vi "Arange_Displays_V2.vi"(0 "Display References":refnum<vi>[](array[refnum]), 2 "Action":u16(ring) items=["Read", "Write"], 7 "Number of Channels":i32, 11 "Aspect Ratio (h/w)":dbl) -> (8 "Number of Channels OUT":i32)   [LabVIEW 2014]
uses:
  <vilib>/Utility/miscctls.llb/LVPositionTypeDef.ctl
  <vilib>/Utility/miscctls.llb/LVBoundsTypeDef.ctl
panel:
  in  "Display Number":i32=2
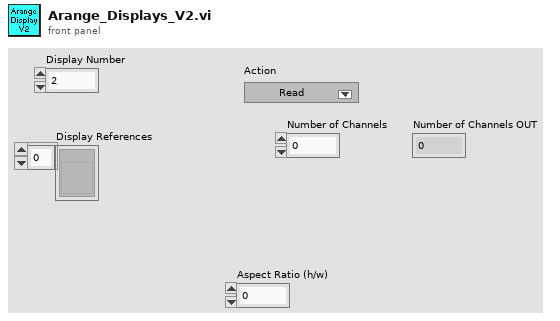
[diagram p1: front panel]
types:
  T1 = typedef "LVPositionTypeDef.ctl" = cluster{"Left":i32, "Top":i32}
  T2 = typedef "LVBoundsTypeDef.ctl" = cluster{"Width":u32, "Height":u32}
  T3 = typedef "LVAllMonitorsDisplayTypeDef.ctl" = cluster{"Bounds":cluster{"Left":i16, "Top":i16, "Right":i16, "Bottom":i16}, "Depth":i16}[]
  T4 = cluster{"Bounds":cluster{"Left":i16, "Top":i16, "Right":i16, "Bottom":i16}, "Depth":i16}
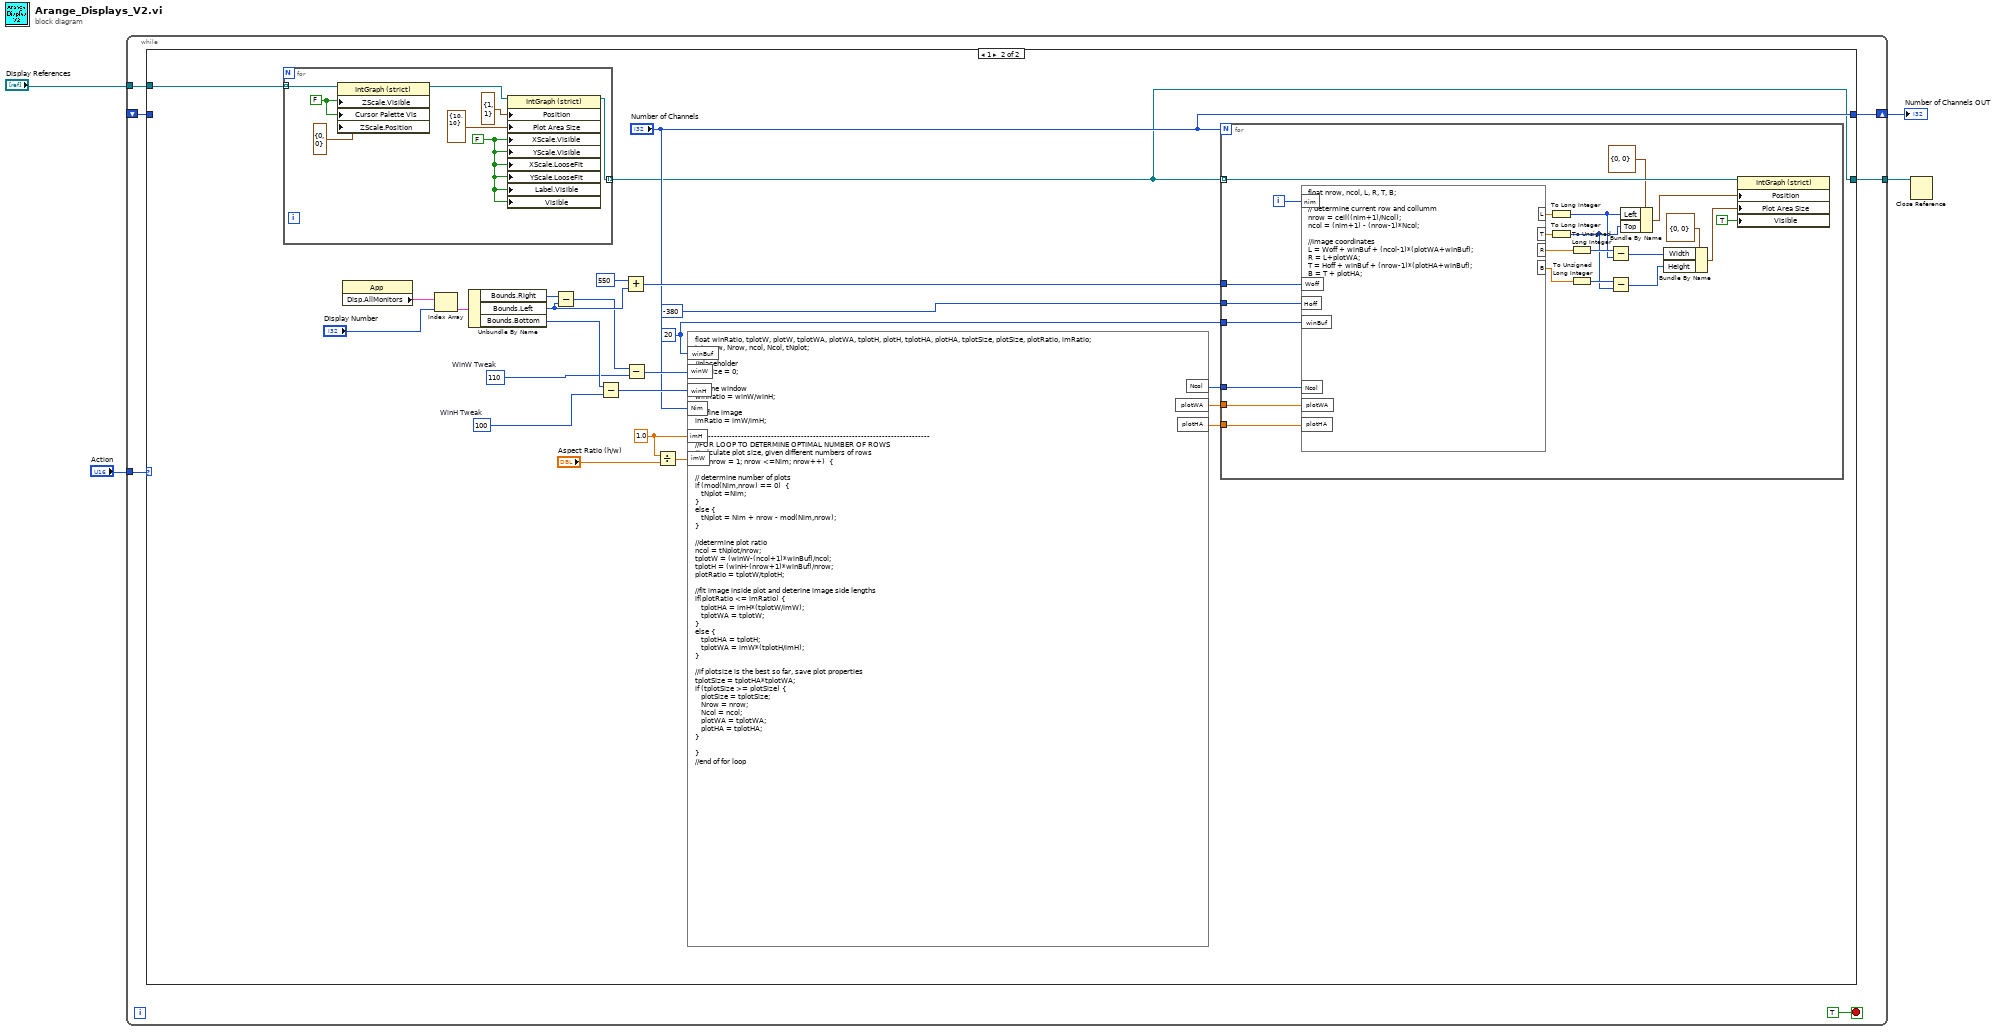
[diagram p0: block diagram]
diagram:
  n1 = while {
    tunnel: "Action" -> [w9]
    shift-right: [w8] -> w3
    shift-left: _ -> [w7]
    tunnel: "Display References" -> [w6]
    tunnel: [w5] -> w1
    stop <- TRUE stop-if-true
    n2 = case shown="1" w9 {
      tunnel: [w12 "Number of Channels"] -> w8
      tunnel: w7 -> [w12 _]
      tunnel: w6 -> [w11 w14]
      tunnel: [w11 w13] -> w5
      frame 0, Default {
      }
      frame 1 {
        w36 = 20 ("WinBuffer")
        w19 = i16 110  # WinW Tweak
        w22 = i16 100  # WinH Tweak
        w16 = 1.0 ("y")
        n3 = for {
          tunnel: [w41] -> w13 mode=indexing
          tunnel: w14 -> [w37] mode=indexing
          w38 = FALSE ("Z Scale.Visible")
          w42 = FALSE ("X Scale.Visible")
          n4 = property class="IntGraph (strict)"(reference=w37, "ZScale.Visible"=w38, "Cursor Palette Vis"=w38, "ZScale.Position"=T1 {"Left"=0, "Top"=0} ("Z Scale.Position")) -> (reference out=w40:refnum<vi>)  [unwired: 1 in, 1 out]
          n5 = property class="IntGraph (strict)"(reference=w40, "Position"=T1 {"Left"=1, "Top"=1}, "Plot Area Size"=T2 {"Width"=10, "Height"=10} ("Plot Area:Size"), "XScale.Visible"=w42, "YScale.Visible"=w42, "XScale.LooseFit"=w42, "YScale.LooseFit"=w42, "Label.Visible"=w42, "Visible"=w42) -> (reference out=w41:refnum<vi>)  [unwired: 1 in, 1 out]
        }
        n6 = property class="App"() -> ("Disp.AllMonitors"=w25:T3)  [unwired: 2 in, 2 out]
        n7 = Index Array(array=w25, index="Display Number") -> (element=w31:T4)
        n8 = Unbundle By Name(w31) -> ("Bounds.Right"=w28:i16, "Bounds.Left"=w27:i16, "Bounds.Bottom"=w24:i16)
        n9 = Subtract(x=w28, y=w27) -> (x-y=w21:i16)
        n10 = Subtract(x=w24, y=w22) -> (x-y=w23:i16)
        n11 = Add(x=i16 550 ("Woff"), y=w27) -> (x+y=w26:i16)
        n12 = Subtract(x=w21, y=w19) -> (x-y=w20:i16)
        n13 = Divide(x=w16, y="Aspect Ratio (h/w)") -> (x/y=w17:dbl)
        n14 = formula code="float winRatio, tplotW, plotW, tplotWA, plotWA, tplotH, plotH, tplotHA, plotHA, tplotSize, plotSize, plotRatio, imRatio;\nint nrow, Nrow, ncol, Ncol, tNplot;\n\n//placeholder\nplotSize = 0;\n\n//define window\nwinRatio = winW/winH;\n\n//define image\nimRatio = imW/imH;\n\n//-----------------------------------------------------------------------------\n//FOR LOOP TO DETERMINE OPTIMAL NUMBER OF ROWS\n//calculate plot size, given different numbers of rows\nfor (nrow = 1; nrow <=Nim; nrow++)  {\n\n// determine number of plots\nif (mod(Nim,nrow) == 0)  {\n   tNplot =Nim;\n}\nelse {\n   tNplot = Nim + nrow - mod(Nim,nrow);\n}\n\n//determine plot ratio\nncol = tNplot/nrow;\ntplotW = (winW-(ncol+1)*winBuf)/ncol;\ntplotH = (winH-(nrow+1)*winBuf)/nrow;\nplotRatio = tplotW/tplotH;\n\n//fit image inside plot and deterine image side lengths\nif(plotRatio <= imRatio) {\n   tplotHA = imH*(tplotW/imW);\n   tplotWA = tplotW;\n}\nelse {\n   tplotHA = tplotH;\n   tplotWA = imW*(tplotH/imH);\n}\n\n//if plotsize is the best so far, save plot properties\ntplotSize = tplotHA*tplotWA;\nif (tplotSize >= plotSize) {\n   plotSize = tplotSize;\n   Nrow = nrow; \n   Ncol = ncol;\n   plotWA = tplotWA;\n   plotHA = tplotHA;\n}\n\n} \n//end of for loop"("winH"=w23, "winW"=w20, "winBuf"=w36, "imW"=w17, "imH"=w16, "Nim"="Number of Channels") -> ("Ncol"=w35:i32, "plotWA"=w34:dbl, "plotHA"=w33:dbl)
        n15 = for {
          N: "Number of Channels" -> [_]
          tunnel: w13 -> [w66] mode=indexing
          tunnel: w36 -> [w65]
          tunnel: w35 -> [w64]
          tunnel: w34 -> [w63]
          tunnel: w33 -> [w62]
          tunnel: -380 ("Hoff") -> [w61]
          tunnel: w26 -> [w60]
          i -> [w67]
          n16 = formula code="float nrow, ncol, L, R, T, B;\n\n// determine current row and collumm\nnrow = ceil((nim+1)/Ncol);\nncol = (nim+1) - (nrow-1)*Ncol;\n\n//Image coordinates\nL = Woff + winBuf + (ncol-1)*(plotWA+winBuf);\nR = L+plotWA;\nT = Hoff + winBuf + (nrow-1)*(plotHA+winBuf);\nB = T + plotHA;"("winBuf"=w65, "Woff"=w60, "Hoff"=w61, "nim"=w67, "Ncol"=w64, "plotWA"=w63, "plotHA"=w62) -> ("L"=w58:dbl, "T"=w57:dbl, "R"=w54:dbl, "B"=w51:dbl)
          n17 = To Long Integer(number=w58) -> (32bit integer=w52:i32)
          n18 = To Long Integer(number=w57) -> (32bit integer=w49:i32)
          n19 = To Unsigned Long Integer(number=w54) -> (unsigned 32bit integer=w53:u32)
          n20 = To Unsigned Long Integer(number=w51) -> (unsigned 32bit integer=w50:u32)
          n21 = Subtract(x=w53, y=w52) -> (x-y=w48:u32)
          n22 = Subtract(x=w50, y=w49) -> (x-y=w47:u32)
          n23 = Bundle By Name(cluster=T1 {"Left"=0, "Top"=0} ("Position"), "Left"=w52, "Top"=w49) -> (w56:T1)
          n24 = Bundle By Name(cluster=T2 {"Width"=0, "Height"=0} ("Plot Area:Size"), "Width"=w48, "Height"=w47) -> (w46:T2)
          n25 = property class="IntGraph (strict)"(reference=w66, "Position"=w56, "Plot Area Size"=w46, "Visible"=TRUE) -> ()  [unwired: 1 in, 2 out]
        }
      }
    }
  }
  "Number of Channels OUT" <- w3
  n26 = Close Reference(reference=w1) -> ()  [unwired: 1 in, 1 out]
